vi "convert units to kg.vi"(9 "sample time (s)":dbl, 10 "Native units":dbl, 11 "Units":string) -> (2 "Mass total (kg)":dbl)   [LabVIEW 2016]
uses:
  Controls/mass flow unit codes.ctl
panel:
  in  "Mass flow units":T1=81 items=["Grams/second"=70, "Grams/minute"=71, "Grams/hour"=72, "Kg/second"=73, "Kg/minute"=74, "Kg/hour"=75, "Kg/day"=76, "Metric tons/minute"=77, "Metric tons/hour"=78, "Metric tons/day"=79, "Pounds/second"=80, "Pounds/minute"=81, "Pounds/hour"=82, "Pounds/day"=83, "Short tons/minute"=84, "Short tons/hour"=85, "Short tons/day"=86, "Long tons/hour"=87, "Long tons/day"=88, "Special"=253]
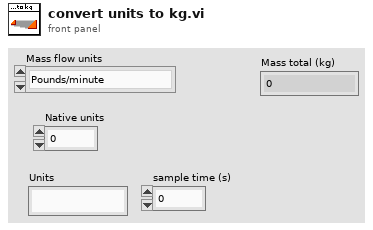
[diagram p1: front panel]
types:
  T1 = typedef "mass flow unit codes.ctl" = u16
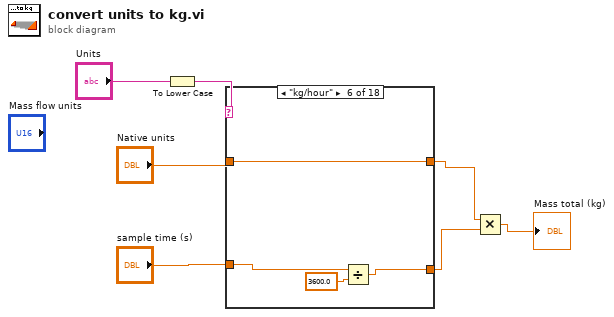
[diagram p0: block diagram]
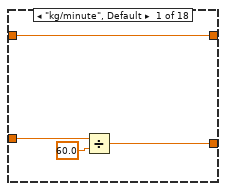
[diagram p2: hidden frame]
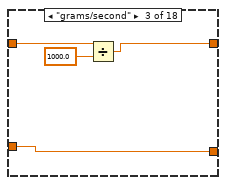
[diagram p4: hidden frame]
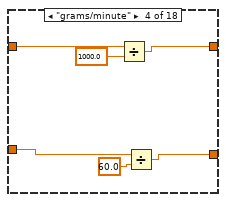
[diagram p5: hidden frame]
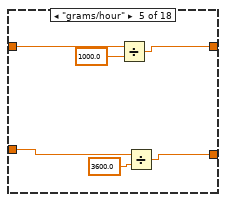
[diagram p6: hidden frame]
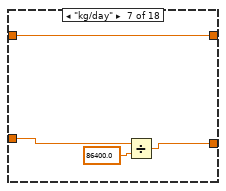
[diagram p7: hidden frame]
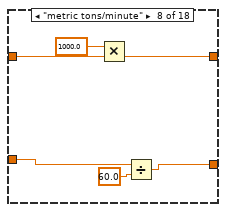
[diagram p8: hidden frame]
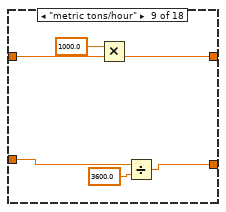
[diagram p9: hidden frame]
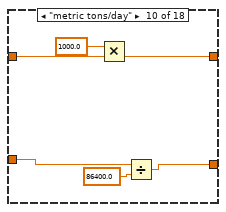
[diagram p10: hidden frame]
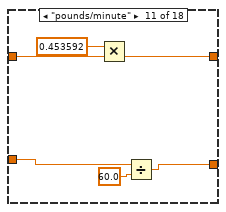
[diagram p11: hidden frame]
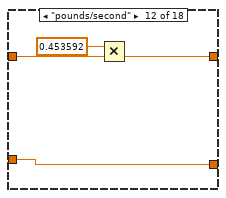
[diagram p12: hidden frame]
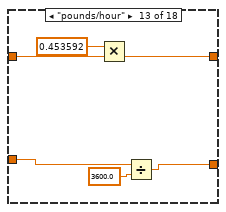
[diagram p13: hidden frame]
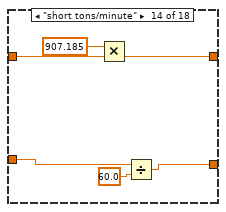
[diagram p14: hidden frame]
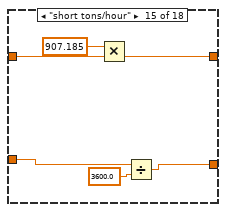
[diagram p15: hidden frame]
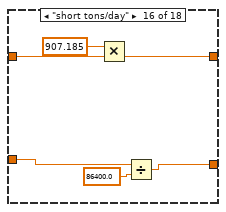
[diagram p16: hidden frame]
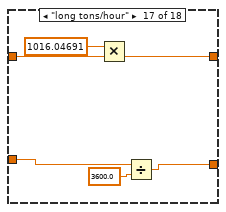
[diagram p17: hidden frame]
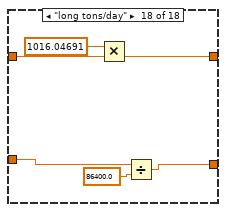
[diagram p18: hidden frame]
diagram:
  n1 = To Lower Case(string="Units") -> (all lower case string=w1:string)
  n2 = case shown="\"kg/hour\"" w1 {
    tunnel: "sample time (s)" -> [w11 w12 w17 w19 w25 w32 w36 w42 w48 w54 w60 w62 w70 w76 w82 w88 w94 w100]
    tunnel: [w9 w12 w17 w18 w24 w31 w35 w41 w47 w53 w59 w62 w69 w75 w81 w87 w93 w99] -> w5
    tunnel: [w8 w13 w14 w21 w27 w30 w34 w39 w45 w51 w57 w64 w67 w73 w79 w85 w91 w97] -> w6
    tunnel: "Native units" -> [w8 w13 w16 w23 w29 w30 w34 w40 w46 w52 w58 w65 w68 w74 w80 w86 w92 w98]
    frame "kg/minute", Default {
      n3 = Divide(x=w11, y=60.0) -> (x/y=w9:dbl)
    }
    frame "kg/second" {
    }
    frame "grams/second" {
      n4 = Divide(x=w16, y=1000.0) -> (x/y=w14:dbl)
    }
    frame "grams/minute" {
      n5 = Divide(x=w23, y=1000.0) -> (x/y=w21:dbl)
      n6 = Divide(x=w19, y=60.0) -> (x/y=w18:dbl)
    }
    frame "grams/hour" {
      n7 = Divide(x=w29, y=1000.0) -> (x/y=w27:dbl)
      n8 = Divide(x=w25, y=3600.0) -> (x/y=w24:dbl)
    }
    frame "kg/hour" {
      n9 = Divide(x=w32, y=3600.0) -> (x/y=w31:dbl)
    }
    frame "kg/day" {
      n10 = Divide(x=w36, y=86400.0) -> (x/y=w35:dbl)
    }
    frame "metric tons/minute" {
      n11 = Multiply(x=1000.0, y=w40) -> (x*y=w39:dbl)
      n12 = Divide(x=w42, y=60.0) -> (x/y=w41:dbl)
    }
    frame "metric tons/hour" {
      n13 = Multiply(x=1000.0, y=w46) -> (x*y=w45:dbl)
      n14 = Divide(x=w48, y=3600.0) -> (x/y=w47:dbl)
    }
    frame "metric tons/day" {
      n15 = Multiply(x=1000.0, y=w52) -> (x*y=w51:dbl)
      n16 = Divide(x=w54, y=86400.0) -> (x/y=w53:dbl)
    }
    frame "pounds/minute" {
      n17 = Multiply(x=0.453592, y=w58) -> (x*y=w57:dbl)
      n18 = Divide(x=w60, y=60.0) -> (x/y=w59:dbl)
    }
    frame "pounds/second" {
      n19 = Multiply(x=0.453592, y=w65) -> (x*y=w64:dbl)
    }
    frame "pounds/hour" {
      n20 = Multiply(x=0.453592, y=w68) -> (x*y=w67:dbl)
      n21 = Divide(x=w70, y=3600.0) -> (x/y=w69:dbl)
    }
    frame "short tons/minute" {
      n22 = Multiply(x=907.185, y=w74) -> (x*y=w73:dbl)
      n23 = Divide(x=w76, y=60.0) -> (x/y=w75:dbl)
    }
    frame "short tons/hour" {
      n24 = Multiply(x=907.185, y=w80) -> (x*y=w79:dbl)
      n25 = Divide(x=w82, y=3600.0) -> (x/y=w81:dbl)
    }
    frame "short tons/day" {
      n26 = Multiply(x=907.185, y=w86) -> (x*y=w85:dbl)
      n27 = Divide(x=w88, y=86400.0) -> (x/y=w87:dbl)
    }
    frame "long tons/hour" {
      n28 = Multiply(x=1016.04691, y=w92) -> (x*y=w91:dbl)
      n29 = Divide(x=w94, y=3600.0) -> (x/y=w93:dbl)
    }
    frame "long tons/day" {
      n30 = Multiply(x=1016.04691, y=w98) -> (x*y=w97:dbl)
      n31 = Divide(x=w100, y=86400.0) -> (x/y=w99:dbl)
    }
  }
  n32 = Multiply(x=w6, y=w5) -> (x*y=→"Mass total (kg)":dbl)
